vi "DigiPattern File Converter.vi"(8 "error in (no error)":errorcluster, 9 "Pattern  Contents":string, 10 "Pattern Name":string, 11 "PinMap":path) -> (0 "error out":errorcluster)   [LabVIEW 2018]
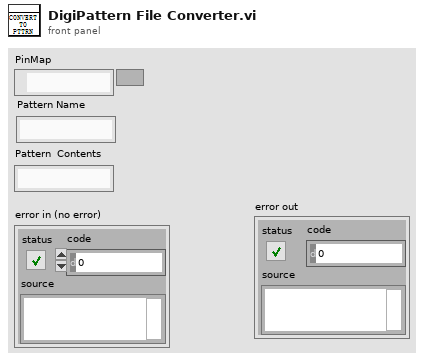
[diagram p1: front panel]
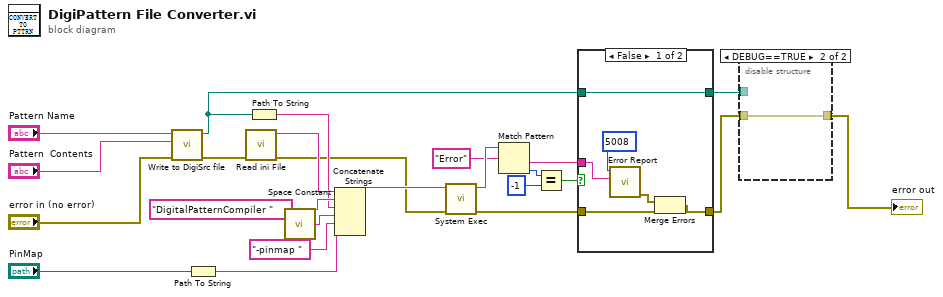
[diagram p0: block diagram]
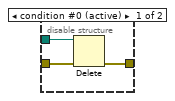
[diagram p2: hidden frame]
diagram:
  n1 = call "Write to DigiSrc file.vi"("error in (no error)"="error in (no error)", "Pattern  Contents"="Pattern  Contents", "Pattern Name"="Pattern Name") -> ("error out"=w19:errorcluster, "DigiSrc File"=w8:path)  [unwired: 7 in]
  n2 = Path To String(path="PinMap") -> (string=w20:string)
  n3 = call "Read ini File.vi"("error in (no error)"=w19) -> ("error out"=w9:errorcluster, "value"=w21:string)  [unwired: 9 in]
  n4 = Path To String(path=w8) -> (string=w18:string)
  n5 = call <vilib>:"Space Constant.vi"() -> ("String"=w23:string)
  n6 = Concatenate Strings(w21, "DigitalPatternCompiler " ("string"), w18, w23, "-pinmap " ("string"), w20) -> (w10:string)
  n7 = call <vilib>:"System Exec.vi"("error in (no error)"=w9, "command line"=w10) -> ("error out"=w11:errorcluster, "standard output"=w17:string)  [unwired: 6 in, 2 out]
  n8 = Match Pattern(string=w17, regular expression="Error") -> (after substring=w12:string, offset past match=w15:i32)  [unwired: 1 in, 2 out]
  n9 = Equal?(x=w15, y=-1) -> (x = y?=w13:bool)
  n10 = case shown="False" w13 {
    tunnel: w12 -> [w26 _]
    tunnel: w11 -> [w30 w32]
    tunnel: [w29 w32] -> w2
    tunnel: w8 -> [w28 w31]
    tunnel: [w28 w31] -> w7
    frame False {
      n11 = call "Error Report.vi"("Additional info"=w26, "Error Code"=i16 5008) -> ("error out"=w25:errorcluster)  [unwired: 9 in]
      n12 = Merge Errors(w25, w30) -> (w29:errorcluster)
    }
    frame True {
    }
  }
  n13 = disable-structure shown="DEBUG==TRUE" {
    disable-tunnel: [w35 w36] -> w1
    disable-tunnel: w7 -> [w34 _]
    disable-tunnel: w2 -> [w33 w36]
    frame condition #0 (active) {
      n14 = Delete(path (use dialog)=w34, error in=w33) -> (error out=w35:errorcluster)  [unwired: 3 in, 2 out]
    }
    frame condition #1 {
    }
  }
  "error out" <- w1
